vi "Run Script.vi"(8 "error in (no error)":errorcluster caption="错误输入（无错误）", 11 "2601B 输入":refnum<class "2601B.lvclass">) -> (0 "error out":errorcluster caption="错误输出", 3 "2601B 输出":refnum<class "2601B.lvclass">)   [LabVIEW 2020, in "2601B.lvclass"]
uses:
  2601B.lvclass
  2601B.lvclass/2601B.ctl
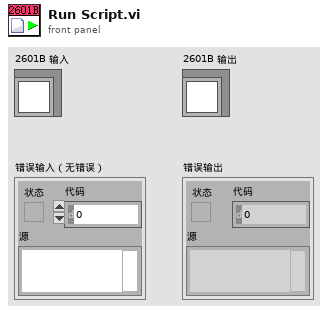
[diagram p1: front panel]
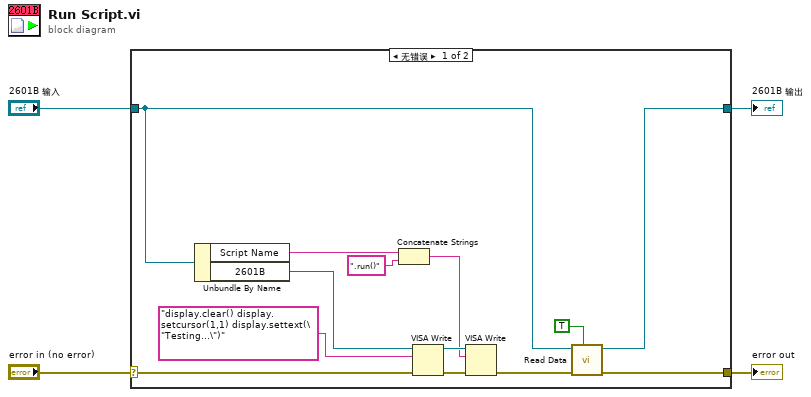
[diagram p0: block diagram]
diagram:
  n1 = case shown="无错误" "error in (no error)" {
    selector: "error in (no error)" -> [w17 w19]
    tunnel: [w11 w19] -> w3
    tunnel: [w10 w18] -> w1
    tunnel: "2601B 输入" -> [w9 w18]
    frame No Error {
      n2 = Unbundle By Name(w9) -> ("Script Name"=w5:string, "2601B"=w15:refnum<visa-resource-name>)
      n3 = Concatenate Strings(w5, ".run()" ("string")) -> (w7:string)
      n4 = VISA Write(VISA resource name=w15, write buffer="display.clear() display.setcursor(1,1) display.settext(\"Testing...\")", error in (no error)=w17) -> (VISA resource name out=w12:refnum<visa-resource-name>, error out=w16:errorcluster)  [unwired: 1 out]
      n5 = VISA Write(VISA resource name=w12, write buffer=w7, error in (no error)=w16) -> (error out=w13:errorcluster)  [unwired: 2 out]
      n6 = call "Read Data.vi"("初始化?"=TRUE, "error in (no error)"=w13, "2601B 输入"=w9) -> ("error out"=w11:errorcluster, "2601B 输出"=w10:refnum<class "2601B.lvclass">)  [unwired: 5 in, 2 out]
    }
    frame Error {
    }
  }
  "error out" <- w3
  "2601B 输出" <- w1
